vi "DB Tools Execute Query.vi"   [LabVIEW 2017, in "NI_Database_API.lvlib"]
doc: "Executes an SQL query and returns a recordset reference that you must eventually free with the DB Tools Free Object VI. Wire data to the reference input to determine the polymorphic instance to use or manually select the instance."
uses:
  <vilib>/addons/database/NI_Database_API.lvlib
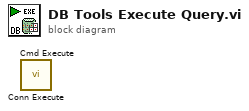
[diagram p0: block diagram]
diagram:
  n1 = call <vilib>:"Conn Execute.vi"() -> ()  [unwired: 8 in, 2 out]
  n2 = call <vilib>:"Cmd Execute.vi"() -> ()  [unwired: 8 in, 2 out]
